vi "Begin.vi"(8 "error in":errorcluster) -> (0 "error out":errorcluster)   [LabVIEW 2017]
doc: "Called before other user functions, this VI is expected to open initial I/O refnums, load in file data, and do all program initialization. Notice that the <B>error out</B> terminal is simply used for data flow. Wiring it to other structures or subVIs ensures that this VI runs first."
uses:
  <vilib>/Rock Robotics/WPI/SafetyOutput/WPI_SafetyOutputConfigMenu.ctl
  <vilib>/Rock Robotics/WPI/DriverStation/WPI_DriverStationRobotMode2.ctl
  <vilib>/Rock Robotics/WPI/Joystick/WPI_JoystickDeviceEnum.ctl
  <vilib>/Rock Robotics/WPI/ThirdParty/Phoenix-LabVIEW/Motor Controller/Controls/CTRE_Phoenix_MotorControl_ControlMode.ctl
  <vilib>/Rock Robotics/WPI/ThirdParty/Phoenix-LabVIEW/Motor Controller/Controls/CTRE_Phoenix_MotorControl_NeutralMode.ctl
  <vilib>/Rock Robotics/WPI/ThirdParty/Phoenix-LabVIEW/Motor Controller/Controls/CTRE_Phoenix_MotorControl_FeedbackDevice.ctl
  Robot Global Data.vi
  <vilib>/Rock Robotics/Network Tables/NT Write String Array.vi
  <vilib>/Rock Robotics/WPI/RobotDrive/WPI_RobotDriveOpen2MotorWithExistingMotors.vi
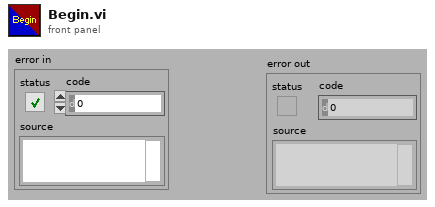
[diagram p1: front panel]
types:
  T1 = typedef "CTRE_Phoenix_MotorControl_ControlMode.ctl" = u16
  T2 = typedef "CTRE_Phoenix_MotorControl_FeedbackDevice.ctl" = i8
  T3 = typedef "CTRE_Phoenix_MotorControl_NeutralMode.ctl" = enum8{"EEPROMSetting", "Override to Coast", "Override to Brake"}
  T4 = typedef "WPI_JoystickDeviceEnum.ctl" = enum16{"USB 0", "USB 1", "USB 2", "USB 3", "USB 4", "USB 5"}
  T5 = typedef "WPI_DriverStationRobotMode2.ctl" = enum16{"Autonomous Disabled", "Autonomous Enabled", "Teleop Disabled", "Teleop Enabled", "Disconnected", "Finish", "Test Disabled", "Test Enabled", "Emergency Stopped"}
  T6 = typedef "WPI_SafetyOutputConfigMenu.ctl" = enum16{"Enable", "Disable"}
  T7 = typedef "WPI_JoystickDevRef.ctl" = cluster{"Device":T4}
  T8 = typedef "WPI_MotorControlDeviceRef.ctl" = cluster{"DeviceStatus":errorcluster, "Type":T9, "PWM":cluster{"PWM Channel":T10, "DeadBand":T11}, "CAN":cluster{"Device Number":u8, "SetOutput VI Ref":variant, "GetOutput VI Ref":variant, "Enable VI Ref":variant, "Disable VI Ref":variant, "Data":variant}, "Invert":bool, "DIO PWM":cluster{"PWM \"Enable\" Channel":T10, "DIOChannel":T12, "PWM Rate":dbl}}
  T9 = typedef "WPI_MotorControlType.ctl" = enum16{"PWM", "CAN", "DIO PWM"}
  T10 = typedef "FPGA_DIOPWMChannel.ctl" = enum8{"PWM 0", "PWM 1", "PWM 2", "PWM 3", "PWM 4", "PWM 5", "PWM 6", "PWM 7", "PWM 8", "PWM 9", "PWM MXP 0", "PWM MXP 1", "PWM MXP 2", "PWM MXP 3", "PWM MXP 4", "PWM MXP 5", "PWM MXP 6", "PWM MXP 7", "PWM MXP 8", "PWM MXP 9", "Invalid"}
  T11 = typedef "WPI_PWMDeadband.ctl" = cluster{"Name":string, "maxPositivePwm":i32, "minPositivePwm":i32, "centerPwm":i32, "maxNegativePwm":i32, "minNegativePwm":i32, "angularRange":u16}
  T12 = typedef "FPGA_DIOChannel.ctl" = enum8{"DIO 0", "DIO 1", "DIO 2", "DIO 3", "DIO 4", "DIO 5", "DIO 6", "DIO 7", "DIO 8", "DIO 9", "DIO MXP 0", "DIO MXP 1", "DIO MXP 2", "DIO MXP 3", "DIO MXP 4", "DIO MXP 5", "DIO MXP 6", "DIO MXP 7", "DIO MXP 8", "DIO MXP 9", "DIO MXP 10", "DIO MXP 11", "DIO MXP 12", "DIO MXP 13", "DIO MXP 14", "DIO MXP 15", "SPI Port CS1", "SPI Port CS2", "SPI Port CS3", "SPI Port MISO", "SPI Port MOSI", "Invalid"}
  T13 = typedef "WPI_RobotDriveDevRef.ctl" = cluster{"DevStatus":errorcluster, "Motors[]":T8[], "Square Inputs":bool, "Max Output":dbl}
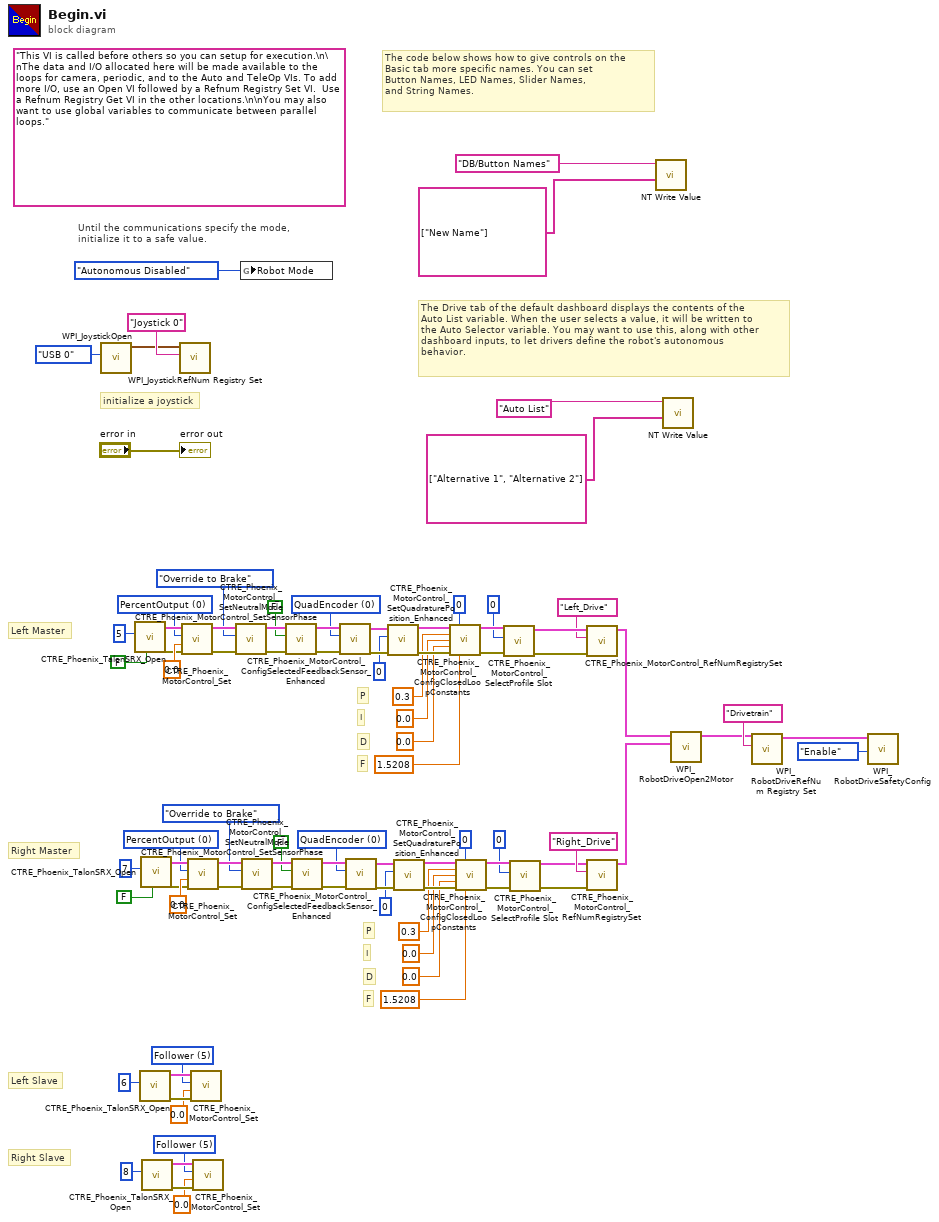
[diagram p0: block diagram]
diagram:
  w6 = T1 5 items=["PercentOutput"=0, "Position"=1, "Velocity"=2, "Current"=3, "Follower"=5, "MotionProfile"=6, "MotionMagic"=7, "MotionMagicArc"=8, "MotionProfileArc"=10, "Disabled"=15] ("Control Mode")
  w10 = T1 5 items=["PercentOutput"=0, "Position"=1, "Velocity"=2, "Current"=3, "Follower"=5, "MotionProfile"=6, "MotionMagic"=7, "MotionMagicArc"=8, "MotionProfileArc"=10, "Disabled"=15] ("Control Mode")
  w34 = T2 0 items=["None"=-1, "QuadEncoder"=0, "Analog"=2, "Tachometer"=4, "Pulse Width Encoded Position"=8, "Sensor Sum (S0 + S1)"=9, "Sensor Difference (D0 - D1)"=10, "Remote Source 0"=11, "Remote Source 1"=12, "Software Emulated"=15] ("Feedback Device")
  w45 = T1 0 items=["PercentOutput"=0, "Position"=1, "Velocity"=2, "Current"=3, "Follower"=5, "MotionProfile"=6, "MotionMagic"=7, "MotionMagicArc"=8, "MotionProfileArc"=10, "Disabled"=15] ("Control Mode")
  w61 = T2 0 items=["None"=-1, "QuadEncoder"=0, "Analog"=2, "Tachometer"=4, "Pulse Width Encoded Position"=8, "Sensor Sum (S0 + S1)"=9, "Sensor Difference (D0 - D1)"=10, "Remote Source 0"=11, "Remote Source 1"=12, "Software Emulated"=15] ("Feedback Device")
  w72 = T1 0 items=["PercentOutput"=0, "Position"=1, "Velocity"=2, "Current"=3, "Follower"=5, "MotionProfile"=6, "MotionMagic"=7, "MotionMagicArc"=8, "MotionProfileArc"=10, "Disabled"=15] ("Control Mode")
  (unwired) "This VI is called before others so you can setup for execution.\n\nThe data and I/O allocated here will be made available to the loops for camera, periodic, and to the Auto and TeleOp VIs. To add more I/O, use an Open VI followed by a Refnum Registry Set VI.  Use a Refnum Registry Get VI in the other locations.\n\nYou may also want to use global variables to communicate between parallel loops."
  # "Right Slave"
  # "Left Slave"
  # "Right Master"
  # "Left Master"
  # "F"
  # "D"
  # "I"
  # "P"
  # "F"
  # "D"
  # "I"
  # "P"
  # "The Drive tab of the default dashboard displays the contents of the\nAuto List variable. When the user selects a value, it will be written to\nthe Auto Selector variable. You may want to use this, along with other\ndashboard inputs, to let drivers define the robot's autonomous\nbehavior."
  # "The code below shows how to give controls on the\nBasic tab more specific names. You can set\nButton Names, LED Names, Slider Names,\nand String Names."
  # "initialize a joystick"
  # "Until the communications specify the mode,\ninitialize it to a safe value."
  n1 = call <vilib>:"WPI_JoystickOpen.vi"("JoystickDevice"=WPI_JoystickDeviceEnum."USB 0") -> ("JoystickDevRef"=w82:T7)  [unwired: 10 in]
  n2 = call <vilib>:"CTRE_Phoenix_TalonSRX_Open.vi"("Invert"=FALSE, "Device Number"=u8 5) -> ("error out"=w65:errorcluster, "CAN Talon SRX Ref"=w73:T8)  [unwired: 8 in]
  n3 = call <vilib>:"CTRE_Phoenix_TalonSRX_Open.vi"("Device Number"=u8 6) -> ("error out"=w12:errorcluster, "CAN Talon SRX Ref"=w11:T8)  [unwired: 9 in]
  n4 = call <vilib>:"CTRE_Phoenix_TalonSRX_Open.vi"("Invert"=FALSE, "Device Number"=u8 7) -> ("error out"=w38:errorcluster, "CAN Talon SRX Ref"=w46:T8)  [unwired: 8 in]
  n5 = call <vilib>:"CTRE_Phoenix_TalonSRX_Open.vi"("Device Number"=u8 8) -> ("error out"=w8:errorcluster, "CAN Talon SRX Ref"=w7:T8)  [unwired: 9 in]
  n6 = call <vilib>:"WPI_JoystickRefNum Registry Set.vi"("refnum name"="Joystick 0", "JoystickDevRef"=w82) -> ()  [unwired: 8 in, 2 out]
  n7 = call <vilib>:"CTRE_Phoenix_MotorControl_Set.vi"("error in (no error)"=w65, "Output"=0.0, "Control Mode"=w72, "PhoenixMotorControlDevRef"=w73) -> ("error out"=w66:errorcluster, "PhoenixMotorControlDevRef"=w70:T8)  [unwired: 6 in]
  n8 = call <vilib>:"CTRE_Phoenix_MotorControl_Set.vi"("error in (no error)"=w38, "Output"=0.0, "Control Mode"=w45, "PhoenixMotorControlDevRef"=w46) -> ("error out"=w39:errorcluster, "PhoenixMotorControlDevRef"=w43:T8)  [unwired: 6 in]
  n9 = call <vilib>:"CTRE_Phoenix_MotorControl_Set.vi"("error in (no error)"=w12, "Output"=0.0, "Control Mode"=w10, "PhoenixMotorControlDevRef"=w11) -> ()  [unwired: 6 in, 2 out]
  n10 = call <vilib>:"CTRE_Phoenix_MotorControl_Set.vi"("error in (no error)"=w8, "Output"=0.0, "Control Mode"=w6, "PhoenixMotorControlDevRef"=w7) -> ()  [unwired: 6 in, 2 out]
  n11 = call <vilib>:"CTRE_Phoenix_MotorControl_SetNeutralMode.vi"("error in (no error)"=w66, "Motor Control Neutral Mode"=CTRE_Phoenix_MotorControl_NeutralMode."Override to Brake", "PhoenixMotorControlDevRef"=w70) -> ("error out"=w68:errorcluster, "PhoenixMotorControlDevRef"=w67:T8)  [unwired: 7 in]
  n12 = global write "Robot Global Data.vi" "Robot Mode"(WPI_DriverStationRobotMode2."Autonomous Disabled" ("Robot Mode")) -> ()
  n13 = call <vilib>:"CTRE_Phoenix_MotorControl_SetNeutralMode.vi"("error in (no error)"=w39, "Motor Control Neutral Mode"=CTRE_Phoenix_MotorControl_NeutralMode."Override to Brake", "PhoenixMotorControlDevRef"=w43) -> ("error out"=w41:errorcluster, "PhoenixMotorControlDevRef"=w40:T8)  [unwired: 7 in]
  n14 = call <vilib>:"CTRE_Phoenix_MotorControl_SetSensorPhase.vi"("error in (no error)"=w68, "PhaseSensor"=FALSE, "PhoenixMotorControlDevRef"=w67) -> ("error out"=w63:errorcluster, "PhoenixMotorControlDevRef"=w62:T8)  [unwired: 7 in]
  n15 = call <vilib>:"CTRE_Phoenix_MotorControl_SetSensorPhase.vi"("error in (no error)"=w41, "PhaseSensor"=FALSE, "PhoenixMotorControlDevRef"=w40) -> ("error out"=w36:errorcluster, "PhoenixMotorControlDevRef"=w35:T8)  [unwired: 7 in]
  n16 = call <vilib>:"CTRE_Phoenix_MotorControl_ConfigSelectedFeedbackSensor_Enhanced.vi"("error in (no error)"=w63, "Feedback Device"=w61, "PhoenixMotorControlDevRef"=w62) -> ("error out"=w59:errorcluster, "PhoenixMotorControlDevRef"=w60:T8)  [unwired: 7 in]
  n17 = call <vilib>:"CTRE_Phoenix_MotorControl_ConfigSelectedFeedbackSensor_Enhanced.vi"("error in (no error)"=w36, "Feedback Device"=w34, "PhoenixMotorControlDevRef"=w35) -> ("error out"=w32:errorcluster, "PhoenixMotorControlDevRef"=w33:T8)  [unwired: 7 in]
  n18 = call <vilib>:"CTRE_Phoenix_MotorControl_SetQuadraturePosition_Enhanced.vi"("error in (no error)"=w59, "New Position"=0, "PhoenixMotorControlDevRef"=w60) -> ("error out"=w56:errorcluster, "PhoenixMotorControlDevRef"=w57:T8)  [unwired: 7 in]
  n19 = call <vilib>:"CTRE_Phoenix_MotorControl_SetQuadraturePosition_Enhanced.vi"("error in (no error)"=w32, "New Position"=0, "PhoenixMotorControlDevRef"=w33) -> ("error out"=w29:errorcluster, "PhoenixMotorControlDevRef"=w30:T8)  [unwired: 7 in]
  n20 = call <vilib>:"CTRE_Phoenix_MotorControl_ConfigClosedLoopConstants.vi"("PhoenixMotorControlDevRef"=w57, "slotIdx"=0, "P"=0.3, "I"=0.0, "D"=0.0, "error in (no error)"=w56, "F"=1.5208) -> ("PhoenixMotorControlDevRef"=w49:T8, "error out"=w50:errorcluster)  [unwired: 7 in]
  n21 = call <vilib>:"CTRE_Phoenix_MotorControl_ConfigClosedLoopConstants.vi"("PhoenixMotorControlDevRef"=w30, "slotIdx"=0, "P"=0.3, "I"=0.0, "D"=0.0, "error in (no error)"=w29, "F"=1.5208) -> ("PhoenixMotorControlDevRef"=w22:T8, "error out"=w23:errorcluster)  [unwired: 7 in]
  n22 = call <vilib>:"CTRE_Phoenix_MotorControl_SelectProfile Slot.vi"("error in (no error)"=w50, "slotIdx"=0, "PhoenixMotorControlDevRef"=w49) -> ("error out"=w19:errorcluster, "PhoenixMotorControlDevRef"=w18:T8)  [unwired: 7 in]
  n23 = call <vilib>:"CTRE_Phoenix_MotorControl_SelectProfile Slot.vi"("error in (no error)"=w23, "slotIdx"=0, "PhoenixMotorControlDevRef"=w22) -> ("error out"=w15:errorcluster, "PhoenixMotorControlDevRef"=w16:T8)  [unwired: 7 in]
  n24 = call <vilib>:"CTRE_Phoenix_MotorControl_RefNumRegistrySet.vi"("error in (no error)"=w19, "refnum name"="Left_Drive", "PhoenixMotorControlDevRef"=w18) -> ("PhoenixMotorControlDevRef"=w14:T8)  [unwired: 7 in, 1 out]
  n25 = call <vilib>:"CTRE_Phoenix_MotorControl_RefNumRegistrySet.vi"("error in (no error)"=w15, "refnum name"="Right_Drive", "PhoenixMotorControlDevRef"=w16) -> ("PhoenixMotorControlDevRef"=w13:T8)  [unwired: 7 in, 1 out]
  n26 = call-poly <vilib>:"NT Write Value.vi"("String Array"=string[] ["New Name"], "Name"="DB/Button Names") -> ()  [unwired: 9 in, 1 out]
  n27 = call-poly <vilib>:"NT Write Value.vi"("String Array"=string[] ["Alternative 1", "Alternative 2"], "Name"="Auto List") -> ()  [unwired: 9 in, 1 out]
  n28 = call-poly <vilib>:"WPI_RobotDriveOpen2Motor.vi"("Right Motor Dev Ref"=w13, "Left Motor Dev Ref"=w14) -> ("RobotDriveDevRef"=w75:T13)  [unwired: 8 in, 1 out]
  n29 = call <vilib>:"WPI_RobotDriveRefNum Registry Set.vi"("refnum name"="Drivetrain", "RobotDriveDevRef"=w75) -> ("RobotDriveDevRef"=w86:T13)  [unwired: 2 in, 7 out]
  n30 = call <vilib>:"WPI_RobotDriveSafetyConfig.vi"("mode"=WPI_SafetyOutputConfigMenu."Enable", "RobotDriveDevRef"=w86) -> ()  [unwired: 8 in, 2 out]
  "error out" <- "error in"
